vi "ABB Norma 5000 init.vi"(11 "VT and CT Ratios":T1) -> (0 "norma 5000 parms out":T2)   [LabVIEW 2017]
uses:
  ABB global.vi
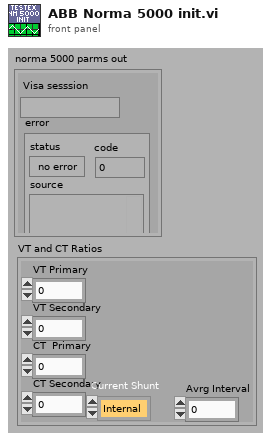
[diagram p1: front panel]
types:
  T1 = cluster{"VT Primary":dbl, "VT Secondary":dbl, "CT  Primary":dbl, "CT Secondary":dbl, "Current Shunt":enum16{"Internal", "External"}, "Avrg Interval":dbl}
  T2 = cluster{"Visa sesssion":refnum<visa-resource-name>, "error":errorcluster}
  T3 = cluster{"Simulate Norma":bool, "Norma 5000 Address":u8, "WebDaq IP Address":string, "Simulate cDAQ":bool}
  T4 = cluster{"dup VISA session":refnum<visa-resource-name>, "error out":errorcluster}
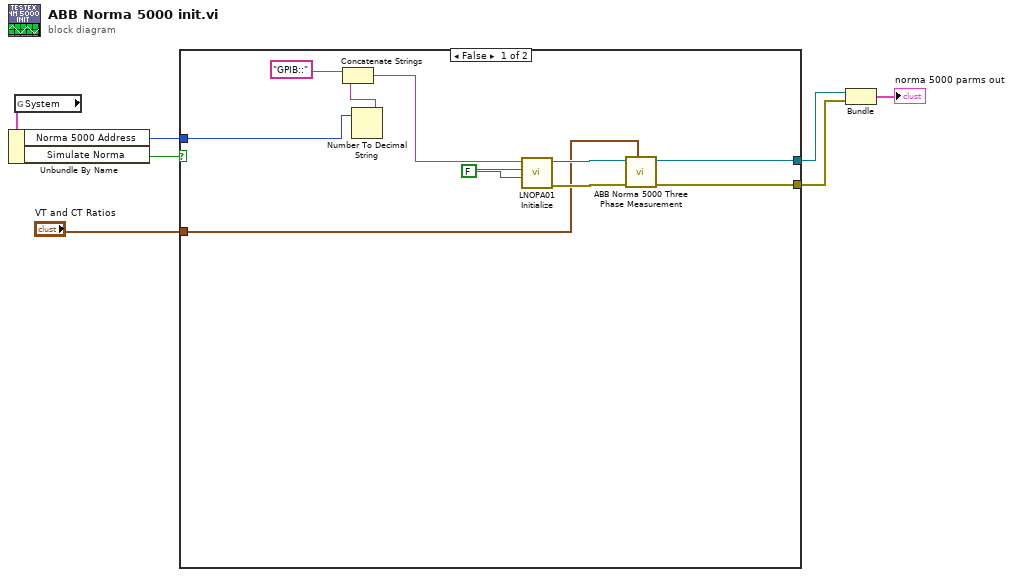
[diagram p0: block diagram]
diagram:
  n1 = global read "ABB global.vi" "System"() -> (w7:T3)
  n2 = Unbundle By Name(w7) -> ("Norma 5000 Address"=w6:u8, "Simulate Norma"=w5:bool)
  n3 = case shown="False" w5 {
    tunnel: w6 -> [w12 _]
    tunnel: [w11 refnum<visa-resource-name> refnum ("dup VISA session")] -> w4
    tunnel: [w10 errorcluster {"status"=FALSE, "code"=0, "source"=""} ("error out")] -> w3
    tunnel: "VT and CT Ratios" -> [w9 _]
    frame False {
      w8 = FALSE ("Reset (T: Reset)")
      n4 = Number To Decimal String(number=w12) -> (decimal integer string=w14:string)  [unwired: 1 in]
      n5 = Concatenate Strings("GPIB::", w14) -> (w13:string)
      n6 = call "LNOPA01 Initialize.vi"("Reset (T: Reset)"=w8, "ID Query (T: Check)"=w8, "Instrument Descriptor (ASRL1::INSTR)"=w13) -> ("error out"=w17:errorcluster, "VISA session"=w16:refnum<visa-resource-name>)  [unwired: 7 in]
      n7 = call "ABB Norma 5000 Three Phase Measurement.vi"("VT and CT Ratios"=w9, "error in (no error)"=w17, "VISA session"=w16) -> ("error out"=w10:errorcluster, "dup VISA session"=w11:refnum<visa-resource-name>)  [unwired: 6 in, 1 out]
    }
    frame True {
      # "Simulate"
    }
  }
  n8 = Bundle("dup VISA session"=w4, "error out"=w3) -> (→"norma 5000 parms out":T4)  [unwired: 1 in]
